vi "IMAQdx Attributes.vi"() -> ()   [LabVIEW 2009, in "HB_IMAQ_Examples.lvlib"]
uses:
  <vilib>/vision/driver/IMAQdx.llb/IMAQdx Attribute Type.ctl
  lib.lib/VisionTools/HGF_VisionTools/IMAQdx_getAttribute_I64.vi
  lib.lib/VisionTools/HGF_VisionTools/IMAQdx_getAttribute_Dbl.vi
  lib.lib/VisionTools/HGF_VisionTools/IMAQdx_getAttribute_Str.vi
  lib.lib/VisionTools/HGF_VisionTools/IMAQdx_getAttribute_Enum.vi
  lib.lib/VisionTools/HGF_VisionTools/IMAQdx_getAttribute_U32.vi
  lib.lib/VisionTools/HGF_VisionTools/IMAQdx_getAttribute_Bool.vi
  lib.lib/VisionTools/HGF_VisionTools/IMAQ_Attribute2Control_Str.vi
  lib.lib/VisionTools/HGF_VisionTools/IMAQ_Attribute2Control_Dbl.vi
  lib.lib/VisionTools/HGF_VisionTools/IMAQ_Attribute2Control_I64.vi
  lib.lib/VisionTools/HGF_VisionTools/IMAQ_Attribute2Control_U32.vi
  lib.lib/VisionTools/HGF_VisionTools/IMAQ_Attribute2Control_Enum.vi
  lib.lib/VisionTools/HGF_VisionTools/IMAQ_Attribute2Control_Bool.vi
  HB_IMAQ_Examples.lvlib
  <vilib>/vision/driver/NI_Vision_Acquisition_Software.lvlib
  lib.lib/VisionTools/HGF_VisionTools/HGF_VisionTools.lvlib
panel:
  out "element":variant
  in  "stop":bool
  in  "Ring":u16(ring) caption="Camera Attributes::Bandwidth::BandwidthControlMode" items=["StreamBytesPerSecond", "SCPD", "Both"]
  out "Boolean":bool caption="Type: Boolean"
  out "String":string caption="Type: Str"
  out "U32":u32 caption="Type: U32" max=0
  out "I64":i64 caption="Type: I64" min=0 max=0
  out "Dbl":dbl caption="Type: Dbl" min=0.0 max=0.0
  in  "Root":string
  out "Attribute Information":T2(array[cluster])
  out "Video Modes":T3(array[cluster])
  out "error out":errorcluster
  out "Camera Information Array":T4(array[cluster]) {"BusType" format="%x"; "SerialNumberLow" format="%.0x"; "SerialNumberHigh" format="%.0x"}
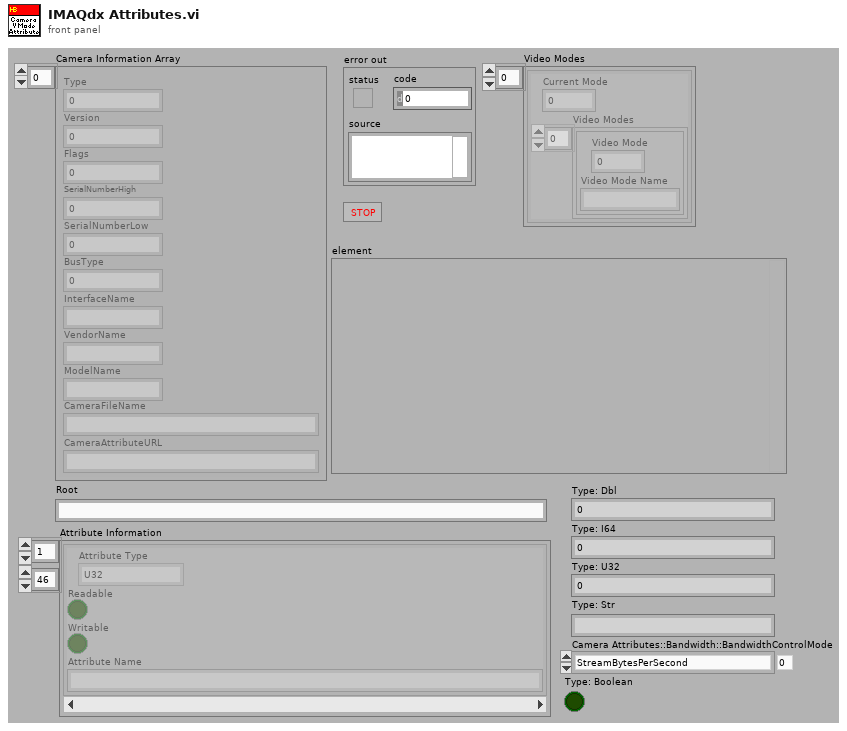
[diagram p1: front panel]
types:
  T1 = typedef "NI_Vision_Acquisition_Software.lvlib/IMAQdx Attribute Type.ctl" = enum32{"U32", "I64", "DBL", "String", "Enum", "Bool", "Command"}
  T2 = cluster{"Attribute Type":T1, "Readable":bool, "Writable":bool, "Attribute Name":string}[][]
  T3 = cluster{"Current Mode":u32, "Video Modes":cluster{"Video Mode":u32, "Video Mode Name":string}[]}[]
  T4 = cluster{"Type":u32, "Version":u32, "Flags":u32, "SerialNumberHigh":u32, "SerialNumberLow":u32, "BusType":u32, "InterfaceName":string, "VendorName":string, "ModelName":string, "CameraFileName":string, "CameraAttributeURL":string}[]
  T5 = typedef "IMAQdx.ctl" = refnum<k21>
  T6 = cluster{"Video Mode":u32, "Video Mode Name":string}[]
  T7 = cluster{"Attribute Type":T1, "Readable":bool, "Writable":bool, "Attribute Name":string}[]
  T8 = cluster{"Current Mode":u32, "Video Modes":cluster{"Video Mode":u32, "Video Mode Name":string}[]}
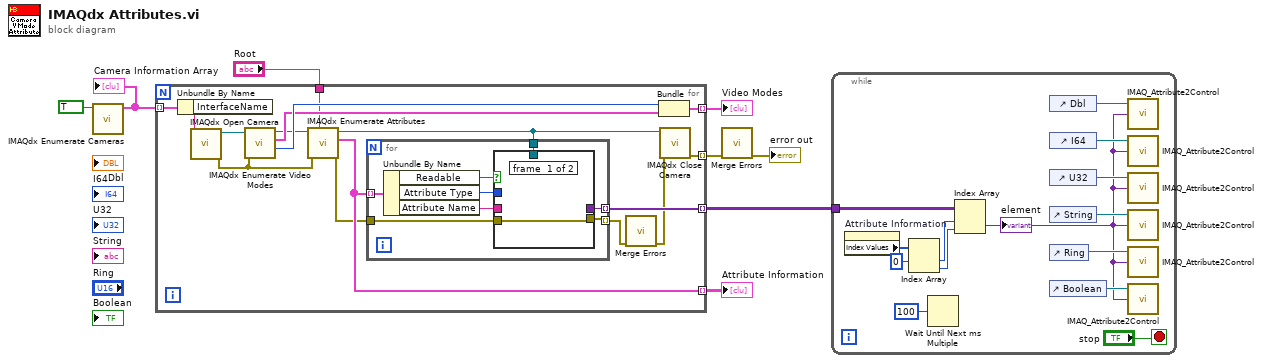
[diagram p0: block diagram]
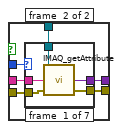
[diagram p2: hidden frame]
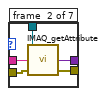
[diagram p3: hidden frame]
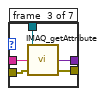
[diagram p4: hidden frame]
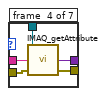
[diagram p5: hidden frame]
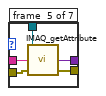
[diagram p6: hidden frame]
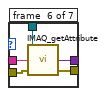
[diagram p7: hidden frame]
diagram:
  n1 = call <vilib>:"IMAQdx Enumerate Cameras.vi"("Connected Only? (Yes)"=TRUE) -> ("Camera Information Array"=w7:T4)  [unwired: 9 in, 1 out]
  "Camera Information Array" <- w7
  n2 = for {
    tunnel: w7 -> [w24] mode=indexing
    tunnel: [w19] -> w6 mode=indexing
    tunnel: [w14] -> w4 mode=indexing
    tunnel: [w18] -> w5 mode=indexing
    tunnel: "Root" -> [w15]
    tunnel: [w12] -> w1 mode=indexing
    n3 = Unbundle By Name(w24) -> ("InterfaceName"=w23:string)
    n4 = call <vilib>:"IMAQdx Open Camera.vi"("Session In"=w23) -> ("error out"=w17:errorcluster, "Session Out"=w16:T5)  [unwired: 9 in]
    n5 = call <vilib>:"IMAQdx Enumerate Video Modes.vi"("error in"=w17, "Session In"=w16) -> ("Current Mode"=w22:u32, "Video Modes"=w21:T6, "Session Out"=w20:T5)  [unwired: 6 in, 1 out]
    n6 = call <vilib>:"IMAQdx Enumerate Attributes.vi"("Root"=w15, "error in"=w17, "Session In"=w20) -> ("error out"=w10:errorcluster, "Attribute Information Array"=w14:T7, "Session Out"=w13:T5)  [unwired: 6 in]
    n7 = for {
      tunnel: w14 -> [w32] mode=indexing
      tunnel: w13 -> [w30]
      tunnel: [w26] -> w12 mode=indexing
      tunnel: w10 -> [w28]
      tunnel: [w27] -> w9 mode=indexing
      n8 = Unbundle By Name(w32) -> ("Readable"=w25:bool, "Attribute Type"=w29:T1, "Attribute Name"=w31:string)
      n9 = case shown="True" w25 {
        tunnel: w31 -> [_ w39]
        tunnel: w30 -> [_ w38]
        tunnel: w29 -> [_ w37]
        tunnel: w28 -> [w33 w36]
        tunnel: [w33 w35] -> w27
        tunnel: [_ w34] -> w26
        frame #0 {
        }
        frame #1 {
          n10 = case shown="\"DBL\"" w37 {
            tunnel: w39 -> [w44 w49 w54 w59 w64 w69 _]
            tunnel: w38 -> [w43 w48 w53 w58 w63 w68 _]
            tunnel: w36 -> [w42 w47 w52 w57 w62 w67 w70]
            tunnel: [w41 w46 w51 w56 w61 w66 w70] -> w35
            tunnel: [w40 w45 w50 w55 w60 w65 _] -> w34
            frame #0 {
              n11 = call-poly "IMAQ_getAttribute.vi"("error in (no error)"=w42, "Attribute Name"=w44, "IMAQdx Session"=w43) -> ("error out"=w41:errorcluster, "IMAQdx Attribute"=w40:variant)  [unwired: 1 out]
            }
            frame #1 {
              n12 = call-poly "IMAQ_getAttribute.vi"("error in (no error)"=w47, "Attribute Name"=w49, "IMAQdx Session"=w48) -> ("error out"=w46:errorcluster, "IMAQdx Attribute"=w45:variant)  [unwired: 1 out]
            }
            frame #2 {
              n13 = call-poly "IMAQ_getAttribute.vi"("error in (no error)"=w52, "Attribute Name"=w54, "IMAQdx Session"=w53) -> ("error out"=w51:errorcluster, "IMAQdx Attribute"=w50:variant)  [unwired: 1 out]
            }
            frame #3 {
              n14 = call-poly "IMAQ_getAttribute.vi"("error in (no error)"=w57, "Attribute Name"=w59, "IMAQdx Session"=w58) -> ("error out"=w56:errorcluster, "IMAQdx Attribute"=w55:variant)  [unwired: 1 out]
            }
            frame #4 {
              n15 = call-poly "IMAQ_getAttribute.vi"("error in (no error)"=w62, "Attribute Name"=w64, "IMAQdx Session"=w63) -> ("error out"=w61:errorcluster, "IMAQdx Attribute"=w60:variant)  [unwired: 1 out]
            }
            frame #5 {
              n16 = call-poly "IMAQ_getAttribute.vi"("error in (no error)"=w67, "Attribute Name"=w69, "IMAQdx Session"=w68) -> ("error out"=w66:errorcluster, "IMAQdx Attribute"=w65:variant)  [unwired: 1 out]
            }
            frame #6 {
            }
          }
        }
      }
    }
    n17 = call <vilib>:"Merge Errors.vi"("error array in"=w9) -> ("error out"=w11:errorcluster)  [unwired: 6 in]
    n18 = Bundle("Current Mode"=w22, "Video Modes"=w21) -> (w18:T8)  [unwired: 1 in]
    n19 = call <vilib>:"IMAQdx Close Camera.vi"("error in"=w11, "Session In"=w13) -> ("error out"=w19:errorcluster)  [unwired: 9 in]
  }
  "Video Modes" <- w5
  "Attribute Information" <- w4
  n20 = call <vilib>:"Merge Errors.vi"("error array in"=w6) -> ("error out"=→"error out":errorcluster)  [unwired: 6 in]
  n21 = while {
    tunnel: w1 -> [w77]
    stop <- "stop" stop-if-true
    n22 = property on="Attribute Information" class="Arr (strict)"() -> ("Index Values"=w71:u32[])  [unwired: 2 in, 2 out]
    n23 = Index Array(array=w71, index #1=0 ("index")) -> (element #1=w75:u32, element #2=w74:u32)  [unwired: 1 in]
    n24 = Wait Until Next ms Multiple(millisecond multiple=u32 100) -> ()  [unwired: 1 out]
    n25 = Index Array(array=w77, index (row)=w75, index (col)=w74) -> (element=w73:variant)
    "element" <- w73
    n26 = control-ref of="Dbl"() -> (w84:refnum<vi>)
    n27 = control-ref of="I64"() -> (w83:refnum<vi>)
    n28 = control-ref of="U32"() -> (w82:refnum<vi>)
    n29 = control-ref of="String"() -> (w81:refnum<vi>)
    n30 = control-ref of="Ring"() -> (w79:refnum<vi>)
    n31 = control-ref of="Boolean"() -> (w80:refnum<vi>)
    n32 = call-poly "IMAQ_Attribute2Control.vi"("IMAQ Attribute"=w73, "Refnum (Dbl)"=w84) -> ()  [unwired: 2 in, 2 out]
    n33 = call-poly "IMAQ_Attribute2Control.vi"("IMAQ Attribute"=w73, "Refnum (I64)"=w83) -> ()  [unwired: 2 in, 2 out]
    n34 = call-poly "IMAQ_Attribute2Control.vi"("IMAQ Attribute"=w73, "Refnum (U32)"=w82) -> ()  [unwired: 2 in, 2 out]
    n35 = call-poly "IMAQ_Attribute2Control.vi"("IMAQ Attribute"=w73, "Refnum (String)"=w81) -> ()  [unwired: 2 in, 2 out]
    n36 = call-poly "IMAQ_Attribute2Control.vi"("IMAQ Attribute"=w73, "Refnum (Enum)"=w79) -> ()  [unwired: 2 in, 2 out]
    n37 = call-poly "IMAQ_Attribute2Control.vi"("IMAQ Attribute"=w73, "Refnum (Boolean)"=w80) -> ()  [unwired: 2 in, 2 out]
  }
